vi "WRP Open Gui.vi"(8 "error in (no error)":errorcluster, 11 "name":string) -> (0 "error out":errorcluster, 3 "function return":i32)   [LabVIEW 2018, in "SesWrapper.lvlib"]
doc: "int STDCALL WRP_SetPropertyDouble(const String property, int index, const double *value);"
uses:
  SesWrapper.lvlib
  build/Debug/SESWrapper.dll
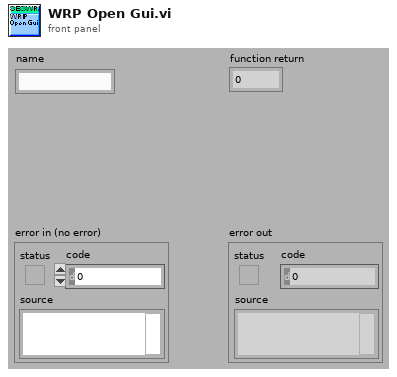
[diagram p1: front panel]
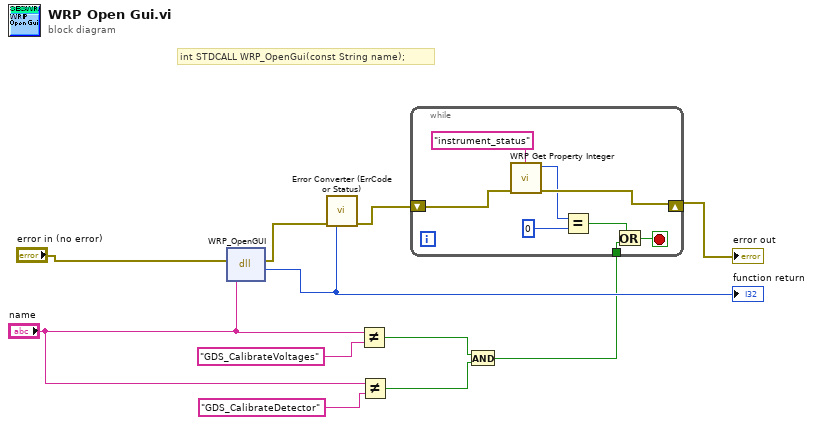
[diagram p0: block diagram]
diagram:
  # "int STDCALL WRP_OpenGui(const String name);"
  n1 = dll-call lib="C:/Development/svn/seswrapper-lib/build/Debug/SESWrapper.*" fn="WRP_OpenGUI" ("SESWrapper.dll:WRP_SetPropertyDouble")(error in="error in (no error)", "name"="name") -> (error out=w10:errorcluster, "return type"=w9:i32)  [unwired: 3 in, 1 out]
  "function return" <- w9
  n2 = call "Error Converter (ErrCode or Status).vi"("error in (no error)"=w10, "error code"=w9) -> ("error out"=w8:errorcluster)  [unwired: 9 in]
  n3 = Not Equal?(x="name", y="GDS_CalibrateVoltages") -> (x != y?=w3:bool)
  n4 = Not Equal?(x="name", y="GDS_CalibrateDetector") -> (x != y?=w2:bool)
  n5 = And(x=w3, y=w2) -> (x .and. y?=w1:bool)
  n6 = while {
    shift-right: [w18] -> w7
    shift-left: w8 -> [w19]
    tunnel: w1 -> [w12]
    stop <- w13 stop-if-true
    n7 = call "WRP Get Property Integer.vi"("error in (no error)"=w19, "property"="instrument_status") -> ("error out"=w18:errorcluster, "value"=w16:i32)  [unwired: 6 in, 2 out]
    n8 = Equal?(x=w16, y=0) -> (x = y?=w14:bool)
    n9 = Or(x=w14, y=w12) -> (x .or. y?=w13:bool)
  }
  "error out" <- w7
